vi "Read Event Registration.vi"(10 "channel":T1) -> (2 "event registration refnums":refnum<event-registration>[](array[refnum]))   [LabVIEW 2019, in "Cmd-Data Event Messenger.lvlib"]
doc: "<p>Reads an <a href=\"nihelplauncher://docs/csh?context=lvcore_lvconcepts_using_events_in_labview\">event registration</a> refnum for an Event Messenger <a href=\"nihelplauncher://docs/csh?context=lvcore_lvconcepts_channel_wires_intro\">channel</a>.</p>"
uses:
  Cmd-Data Event Messenger.lvlib
  ChannelOp.ctl
  ))Channel.ctl
  Event Data.ctl
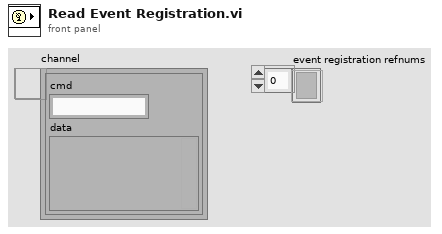
[diagram p1: front panel]
types:
  T1 = typedef "Cmd-Data Event Messenger.lvlib/))Channel.ctl" = refnum<queue>
  T2 = typedef "Cmd-Data Event Messenger.lvlib/ChannelOp.ctl" = enum16{"init", "write", "register", "replicate", "probe"}
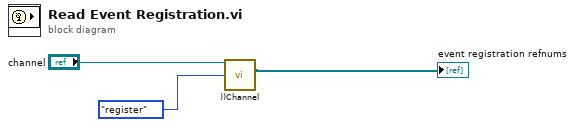
[diagram p0: block diagram]
diagram:
  n1 = call "))Channel.vi"("channel in"="channel", "channelOp"=ChannelOp."register") -> ("event registration refnums"=→"event registration refnums":refnum<event-registration>[])  [unwired: 9 in, 4 out]
